vi "GetSetThermAlarmSettings.vi"(0 "VISA resource name":refnum<visa-resource-name>, 1 "ThermAlarm number":T4 items=["ThermAlarm 1", "ThermAlarm 2", "ThermAlarm 3", "ThermAlarm 4"], 2 "get/set":T5=enum."set", 3 "Input cluster":T2 {"reset" items=["manual reset", "auto reset"]; "delay" min=0 max=30 step=1; "Low Limit" min=0 max=100 step=1; "High Limit" min=0 max=100 step=1; "mute" min=0 max=99 step=1; "warn" min=0 max=99999 step=1}, 5 "error in":errorcluster) -> (14 "VISA resource name out":refnum<visa-resource-name>, 15 "set response":string, 16 "get response":string[](array[string]), 17 "Response cluster":T3, 19 "error out":errorcluster)   [LabVIEW 2023, in "Thermotron 8800.lvlib"]
doc: "AALM\nCommand name: Send or load analog Therm-Alarm settings. NOTE: You must have an original\ntemperature Therm-Alarm and a secondary analog Therm-Alarm installed.\nCommand type: Variable\nDescription: The query command allows you to view the analog information for the Therm-Alarms.\nThe 8800 sends the following response to an AALMn? command:\nSyntax: AALMn? or AALMn, value, low, high, maxex, mute, warn, delay, reset, unused, unused\nWhere n is the Therm-Alarm number. If left blank, the value defaults to 1 (note: actual value sent to 8800 is zero based thus 0-3 for Therm-Alarm 1-4).\nvalue: Analog Therm-Alarm current value\nlow: Analog Therm-Alarm low limit\nhigh: Analog Therm-Alarm high limit\nmaxex: Analog Therm-Alarm maximum excursion\nmute: Analog Therm-Alarm mute time\nwarn: Analog Therm-Alarm warning band\ndelay: Analog Therm-Alarm delay time\nreset: Analog Therm-Alarm reset status (0 = auto reset, 1 = manual reset)\nunused\nunused\n \nThe operation command allows you to set any of the above settings for any analog\nTherm-Alarm hooked up to the chamber. The operation command syntax is as\nfollows:\nAALMn, low, high, mute, warn, delay, reset\nWhere n is the analog Therm-Alarm you wish to set . If left blank, the value\ndefaults to 1 (0 since zero based).\nlow: Analog Therm-Alarm low limit (0 to 100 degrees C)\nhigh: Analog Therm-Alarm high limit (0 to 100 degrees C)\nmute: Analog Therm-Alarm mute time (0 to 99 minutes)\nwarn: Analog Therm-Alarm warning band (0 to 99,999 units)\ndelay: Analog Therm-Alarm delay time (0 to 30 seconds)\nreset: Analog Therm-Alarm reset status (0 = auto reset, 1 = manual reset)\n\nData type: Decimal\nQuery example 1: AALM? (defaults to Therm-Alarm 1)\n8800 response: 10, 0.0,150, 1.5, 10, 12, 15, 0, 0, 0 (The analog Therm-Alarm 0 value is 10, the low limit is 0, the high limit is 150, the maximum excursion is 1.5, the mute time is 10, the warning band is 12, the delay time is 15, the reset status is auto reset\nQuery example 2: AALM3?\n8800 response: 8 (Error code 8 indicates an illegal channel. For more information, see “Error codes”\nlater in this section.)\nOperation example: AALM2,,,,,10,1\n8800 response: 0 (Analog Therm-Alarm 3 (2 is zero based) nuisance delay is set to 10 and the reset is set to auto)"
uses:
  Thermotron 8800.lvlib
  Private/get set.ctl
  Private/ThermAlarmNumberBase0.ctl
  Private/reset.ctl
panel:
  out "CSV response":string
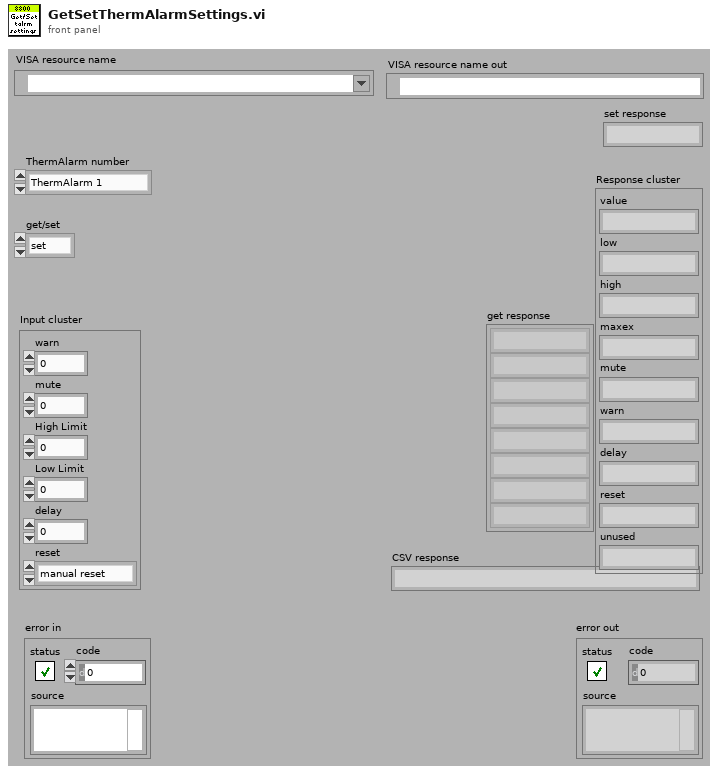
[diagram p1: front panel]
types:
  T1 = typedef "Thermotron 8800.lvlib/reset.ctl" = u16
  T2 = cluster{"warn":i32, "mute":i32, "High Limit":i32, "Low Limit":i32, "delay":i32, "reset":T1}
  T3 = cluster{"value":string, "low":string, "high":string, "maxex":string, "mute":string, "warn":string, "delay":string, "reset":string, "unused":string}
  T4 = typedef "Thermotron 8800.lvlib/ThermAlarmNumberBase0.ctl" = u16
  T5 = typedef "Thermotron 8800.lvlib/get set.ctl" = enum16{"get", "set"}
  T6 = cluster{"appended array[0]":string, "appended array[1]":string, "appended array[2]":string, "appended array[3]":string, "appended array[4]":string, "appended array[5]":string, "appended array[6]":string, "appended array[7]":string, "appended array[8]":string}
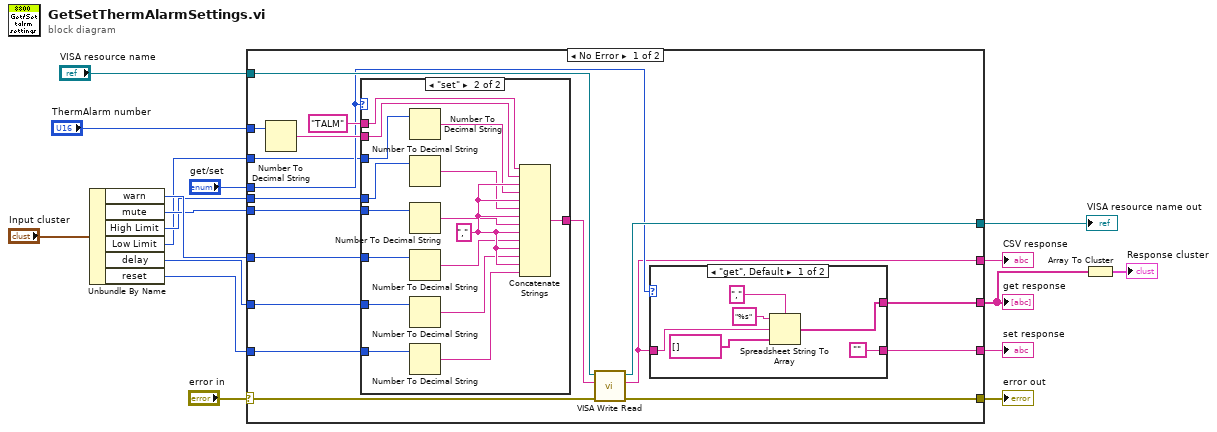
[diagram p0: block diagram]
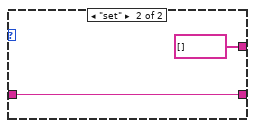
[diagram p2: hidden frame]
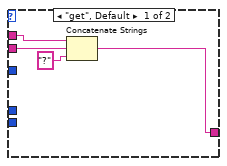
[diagram p3: hidden frame]
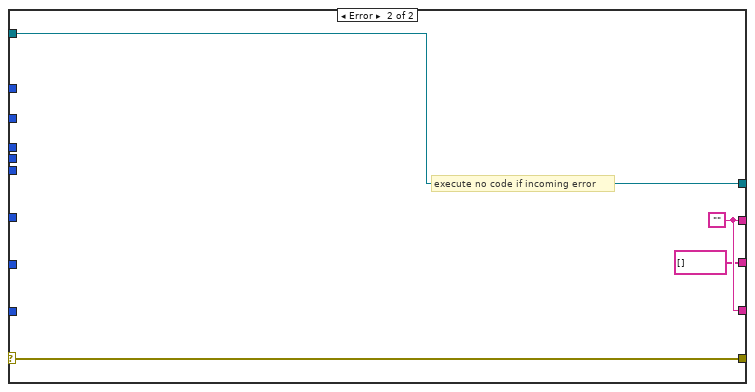
[diagram p4: hidden frame]
diagram:
  n1 = Unbundle By Name("Input cluster") -> ("warn"=w6:i32, "mute"=w5:i32, "High Limit"=w4:i32, "Low Limit"=w3:i32, "delay"=w2:i32, "reset"=w1:T1)
  n2 = case shown="No Error" "error in" {
    selector: "error in" -> [w24 w66]
    tunnel: "VISA resource name" -> [w33 w67]
    tunnel: [w32 w66] -> w16
    tunnel: [w31 w67] -> w15
    tunnel: "get/set" -> [w29 _]
    tunnel: [w28 w65] -> w13
    tunnel: "ThermAlarm number" -> [w27 _]
    tunnel: [w26 w65] -> w11
    tunnel: [w25 string[] [] ("appended array")] -> w9
    tunnel: w3 -> [w23 _]
    tunnel: w4 -> [w22 _]
    tunnel: w5 -> [w21 _]
    tunnel: w6 -> [w20 _]
    tunnel: w2 -> [w19 _]
    tunnel: w1 -> [w18 _]
    frame No Error {
      n3 = Number To Decimal String(number=w27) -> (decimal integer string=w30:string)  [unwired: 1 in]
      n4 = case shown="\"set\"" w29 {
        tunnel: "TALM" ("8800 Command") -> [w46 w63]
        tunnel: [w47 w62] -> w35
        tunnel: w30 -> [w44 w61]
        tunnel: w23 -> [_ w53]
        tunnel: w22 -> [_ w52]
        tunnel: w21 -> [_ w51]
        tunnel: w20 -> [_ w50]
        tunnel: w19 -> [_ w49]
        tunnel: w18 -> [_ w48]
        frame "get", Default {
          n5 = Concatenate Strings(w46, w44, "?" ("8800 Command")) -> (w47:string)
        }
        frame "set" {
          w60 = "," ("string")
          n6 = Number To Decimal String(number=w53) -> (decimal integer string=w59:string)  [unwired: 1 in]
          n7 = Number To Decimal String(number=w52) -> (decimal integer string=w58:string)  [unwired: 1 in]
          n8 = Number To Decimal String(number=w51) -> (decimal integer string=w57:string)  [unwired: 1 in]
          n9 = Number To Decimal String(number=w50) -> (decimal integer string=w56:string)  [unwired: 1 in]
          n10 = Number To Decimal String(number=w49) -> (decimal integer string=w55:string)  [unwired: 1 in]
          n11 = Number To Decimal String(number=w48) -> (decimal integer string=w54:string)  [unwired: 1 in]
          n12 = Concatenate Strings(w63, w61, w60, w59, w60, w58, w60, w57, w60, w56, w60, w55, w60, w54) -> (w62:string)
        }
      }
      n13 = call "VISA Write Read.vi"("error in (no error)"=w24, "8800 Command"=w35, "VISA Refnum in"=w33) -> ("error out"=w32:errorcluster, "read buffer"=w28:string, "VISA Refnum out"=w31:refnum<visa-resource-name>)  [unwired: 6 in]
      n14 = case shown="\"get\", Default" w29 {
        tunnel: w28 -> [w39 w43]
        tunnel: ["" w43] -> w26
        tunnel: [w36 string[] [] ("appended array")] -> w25
        frame "get", Default {
          n15 = Spreadsheet String To Array(delimiter (Tab)=",", format string="%s", spreadsheet string=w39, array type (2D Dbl)=string[] [] ("appended array")) -> (array=w36:string[])
        }
        frame "set" {
        }
      }
    }
    frame Error {
      w65 = ""
      # "execute no code if incoming error"
    }
  }
  "VISA resource name out" <- w15
  "error out" <- w16
  "CSV response" <- w13
  "set response" <- w11
  "get response" <- w9
  n16 = Array To Cluster(array=w9) -> (cluster=→"Response cluster":T6)
